vi "NI-DAQmx.vi"() -> (0 "error out":errorcluster)   [LabVIEW 2017]
uses:
  <vilib>/DAQmx/read.llb/DAQmx Read (Analog 2D DBL NChan NSamp).vi
  Globals/Meas_global.vi
  PWA/PWAtasksGLOBAL.vi
  <vilib>/DAQmx/miscellaneous.llb/DAQmx Fill In Error Info.vi
  <vilib>/DAQmx/configure/timing.llb/DAQmx Timing (Sample Clock).vi
  <vilib>/DAQmx/create/channels.llb/DAQmx Create Channel (AI-Voltage-Basic).vi
  <vilib>/Analysis/baseanly.llb/Mean (DBL).vi
  <resource>/objmgr/daqmx.rc
  <vilib>/Analysis/NI_AALBase.lvlib
panel:
  out "AuditTrail":string[](array[string])
  out "input terminal configuration":i32(ring)=10106 items=["default"=-1, "RSE"=10083, "NRSE"=10078, "Differential"=10106, "Pseudodifferential"=12529]
  out "AI.Voltage.Rngs":dbl[](array[numeric])=[-10.0, 10.0]
  out "TotalSampPerChanAcquired":dbl=1024.0
  out "AvailSampPerChan":u32
  out "CurrReadPos":dbl=1024.0
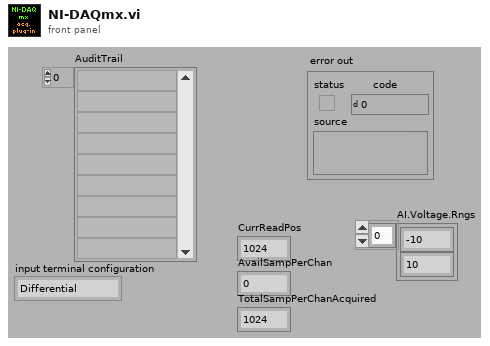
[diagram p1: front panel]
types:
  T1 = typedef "Analysis_info_cluster.ctl" = cluster{"Colour":u32, "Inst type":T2, "Inst name":string, "Symbol":string, "Code name":string, "Extra Info":string, "Inst Array":T3, "Extra Titles":string[], "Extra Values":string[], "U":dbl, "u^2":dbl, "u^3":dbl, "u^4":dbl, "Skew_u":dbl, "Kurt_u":dbl, "Sd Error in Mean":dbl, "% u'/U":dbl, "X":dbl, "Y":dbl, "Z":dbl, "Timescale integral Estimate":dbl, "Sd Error in Variance":dbl, "Calib File":path, "Calib Constants":dbl[], "Output Position":bool, "Full Stats":bool, "Av Sampling Rate":dbl, "Av No of Samples":dbl, "Total Meas Time (s)":dbl, "ADAM Ch Name":string, "Max value":dbl, "Min value":dbl, "Req Sample Rate Hz":dbl, "Sync Delay Time (s)":dbl, "Ch No":i16, "Device ID":string, "Use Latest Calib":bool}
  T2 = typedef "Inst_type.ctl" = enum16{"Propeller anemometer", "Raw voltage", "Pressure Transducer", "Pitot-static tube", "Preston tube", "Hot wire", "Cross wire 1", "Cross wire 2", "Generic Linear", "Generic Polynomial", "Generic BackPoly", "Fast FID", "Thermocouple", "Cold wire", "Pulsed Wire", "LDA Vel", "LDA Tran time", "LDA Arr time", "Microphone"}
  T3 = typedef "Instrument_Array.ctl" = enum16{"PWA", "LDA", "Analogue"}
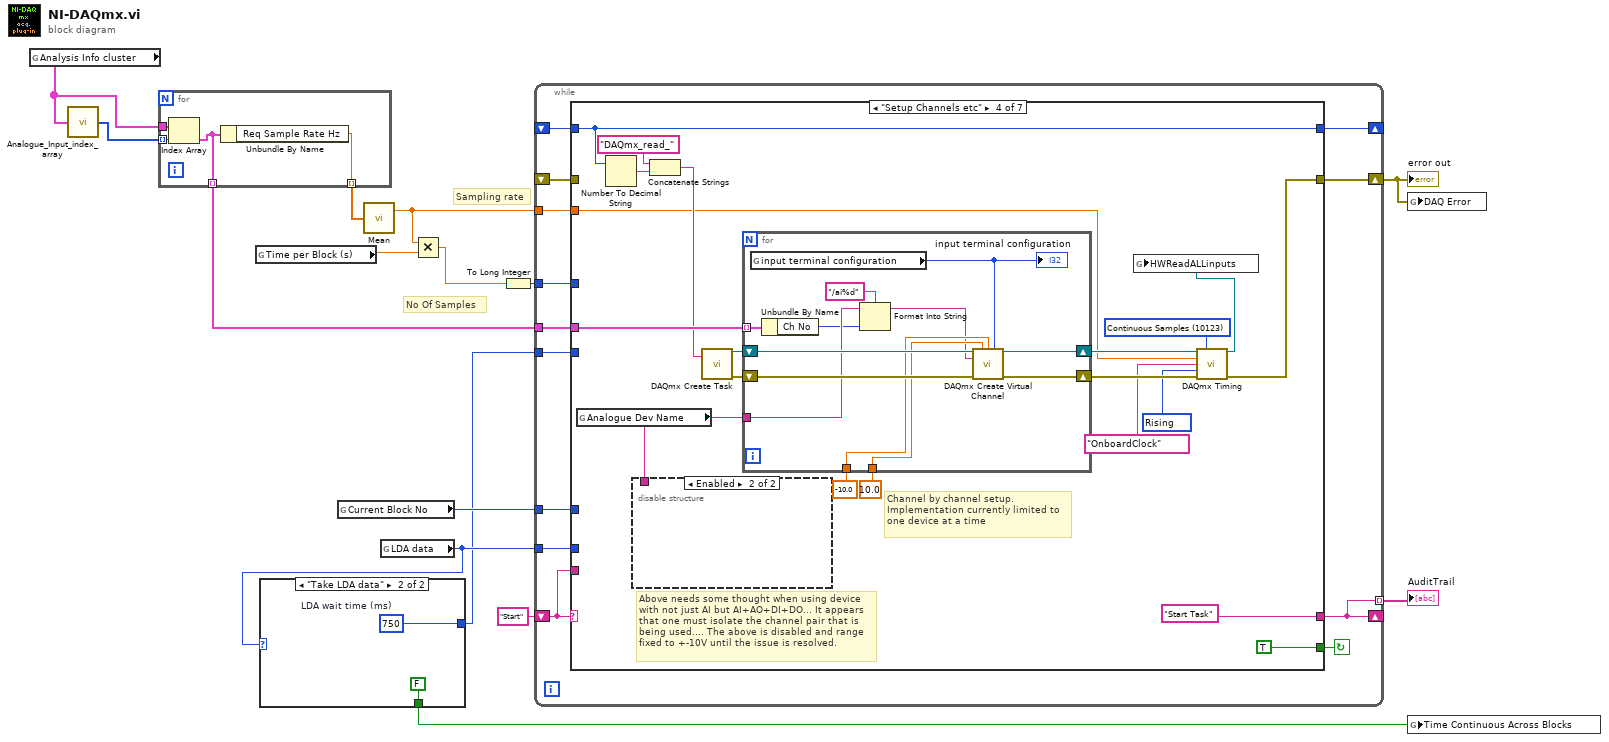
[diagram p0: block diagram]
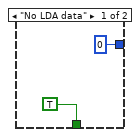
[diagram p2: hidden frame]
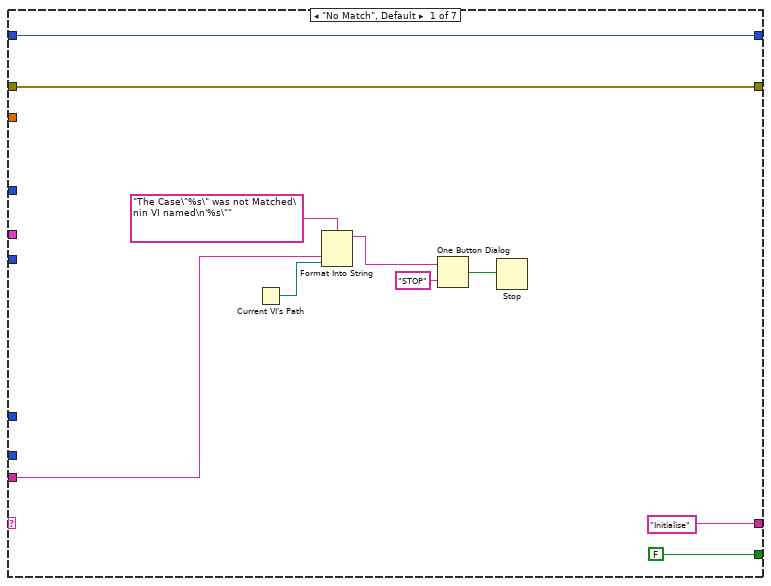
[diagram p3: hidden frame]
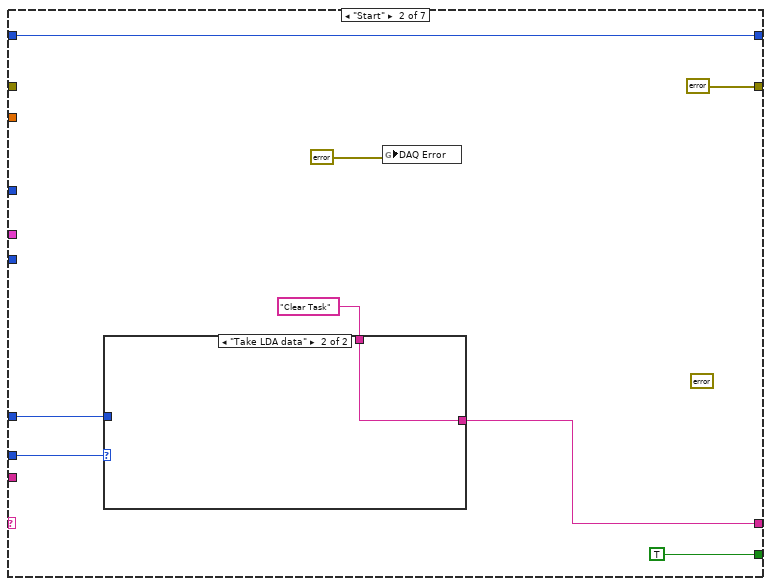
[diagram p4: hidden frame]
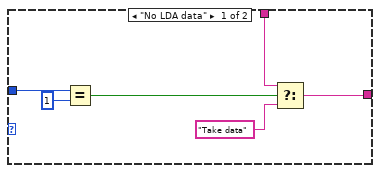
[diagram p5: hidden frame]
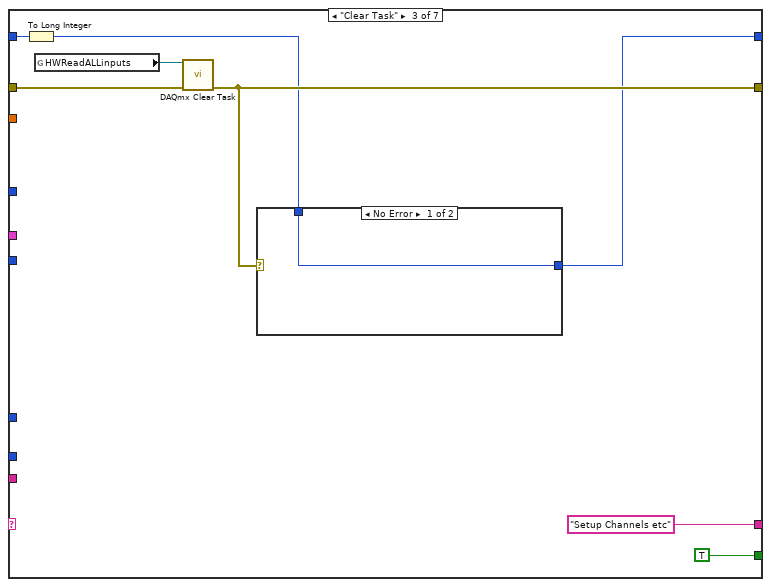
[diagram p6: hidden frame]
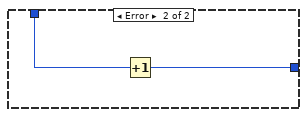
[diagram p7: hidden frame]
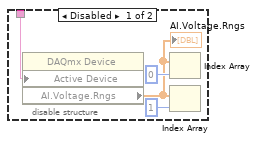
[diagram p8: hidden frame]
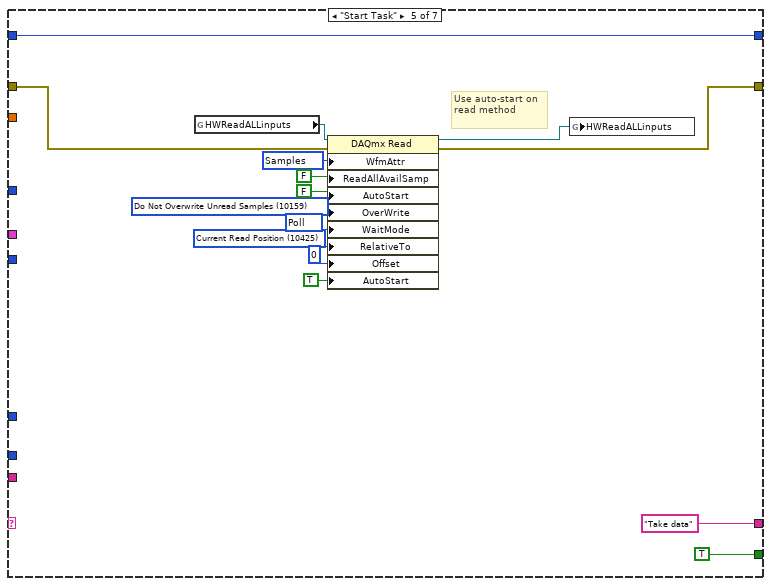
[diagram p9: hidden frame]
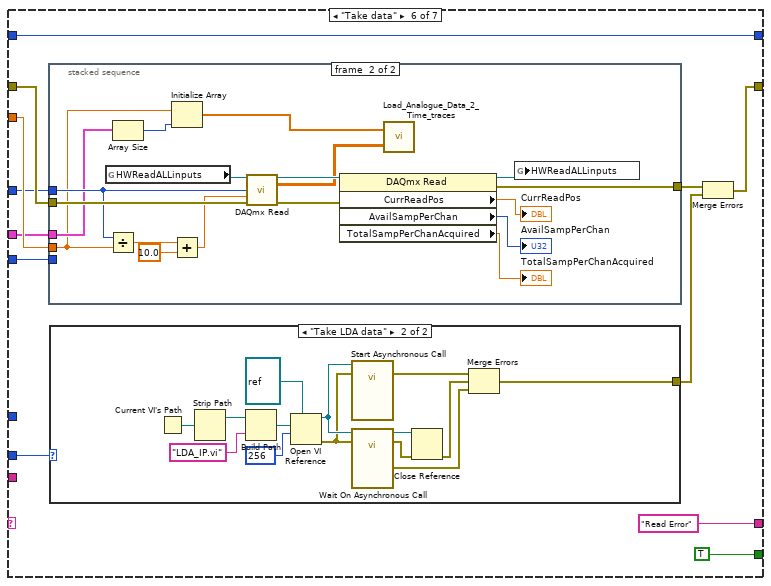
[diagram p10: hidden frame]
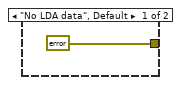
[diagram p11: hidden frame]
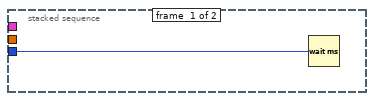
[diagram p12: hidden frame]
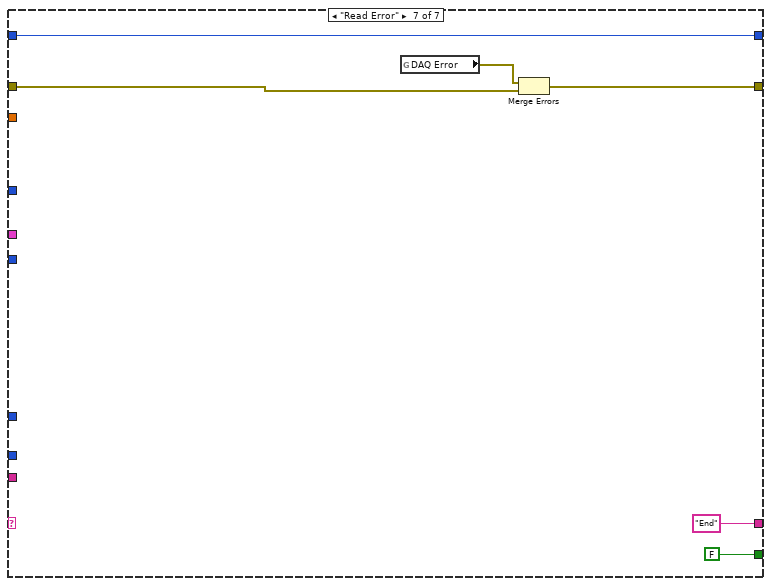
[diagram p13: hidden frame]
diagram:
  # "Sampling rate"
  # "No Of Samples"
  n1 = global read "Meas_global.vi" "Analysis Info cluster"() -> (w7:T1[])
  n2 = call "Analogue_Input_index_array.vi"("Analysis Info cluster"=w7) -> ("Array"=w2:i32[])
  n3 = for {
    tunnel: w7 -> [w19]
    tunnel: w2 -> [w18] mode=indexing
    tunnel: [w17] -> w6 mode=indexing
    tunnel: [w16] -> w1 mode=indexing
    n4 = Index Array(array=w19, index=w18) -> (element=w16:T1)
    n5 = Unbundle By Name(w16) -> ("Req Sample Rate Hz"=w17:dbl)
  }
  n6 = global read "Meas_global.vi" "Time per Block (s)"() -> (w5:dbl)
  n7 = global read "Meas_global.vi" "Current Block No"() -> (w14:i32)
  n8 = call-poly <vilib>:"Mean.vi"("X"=w6) -> ("mean"=w4:dbl)  [unwired: 1 out]
  n9 = global read "Meas_global.vi" "LDA data"() -> (w13:enum16{"No LDA data", "Take LDA data"})
  n10 = case shown="\"Take LDA data\"" w13 {
    tunnel: [TRUE ("Time Continuous across Blocks") FALSE ("Time Continuous across Blocks")] -> w10
    tunnel: [u32 0 ("LDA wait time (ms)") w22] -> w9
    frame "No LDA data" {
    }
    frame "Take LDA data" {
      w22 = u32 750  # LDA wait time (ms)
    }
  }
  n11 = Multiply(x=w4, y=w5) -> (x*y=w3:dbl)
  n12 = To Long Integer(number=w3) -> (32bit integer=w12:i32)
  n13 = while {
    shift-left: "Start" -> [w35]
    shift-right: [w25] -> _
    shift-right: [w29] -> w8
    shift-left: _ -> [w34]
    tunnel: w4 -> [w33]
    tunnel: w12 -> [w32]
    tunnel: w14 -> [w31]
    tunnel: w1 -> [w30]
    shift-right: [w28] -> _
    shift-left: _ -> [w27]
    tunnel: w13 -> [w26]
    tunnel: [w25] -> w11 mode=indexing
    tunnel: w9 -> [w24]
    stop <- w36 continue-if-true
    n14 = case shown="\"Setup Channels etc\"" w35 {
      tunnel: [FALSE TRUE TRUE TRUE TRUE TRUE FALSE] -> w36
      tunnel: ["Initialise" w52 "Setup Channels etc" "Start Task" "Take data" "Read Error" "End" ("f")] -> w25
      tunnel: w35 -> [w41 _ _ _ _ _ _]
      tunnel: [w38 errorcluster {"status"=FALSE, "code"=0, "source"=""} ("error out") w65 w86 w110 w125 w173] -> w29
      tunnel: w34 -> [w38 _ w66 _ w122 w135 w174]
      tunnel: w33 -> [_ _ _ w75 _ w131 _]
      tunnel: w32 -> [_ _ _ _ _ w130 _]
      tunnel: w31 -> [_ w49 _ _ _ _ _]
      tunnel: w30 -> [_ _ _ w85 _ w124 _]
      tunnel: [w37 w51 w64 w74 w120 w132 w172] -> w28
      tunnel: w27 -> [w37 w51 w63 w74 w120 w132 w172]
      tunnel: w26 -> [_ w48 _ _ _ w128 _]
      tunnel: w24 -> [_ _ _ _ _ w129 _]
      frame "No Match", Default {
        n15 = Current VI's Path() -> (path=w40:path)
        n16 = Format Into String(format string="The Case\"%s\" was not Matched\nin VI named\n'%s\"" ("Format String"), w41, w40) -> (resulting string=w44:string)  [unwired: 2 in, 1 out]
        n17 = One Button Dialog(message=w44, button name ("OK")="STOP") -> (true=w42:bool)
        n18 = Stop(stop? (T)=w42) -> ()
      }
      frame "Start" {
        (unwired) errorcluster {"status"=FALSE, "code"=0, "source"=""} ("error out")
        n19 = case shown="\"Take LDA data\"" w48 {
          tunnel: "Clear Task" -> [w60 w61]
          tunnel: [w58 w61] -> w52
          tunnel: w49 -> [w57 _]
          frame "No LDA data" {
            n20 = Equal?(x=w57, y=1) -> (x = y?=w55:bool)
            n21 = Select(t=w60, s=w55, f="Take data") -> (s? t:f=w58:string)
          }
          frame "Take LDA data" {
          }
        }
        n22 = global write "Meas_global.vi" "DAQ Error"(errorcluster {"status"=FALSE, "code"=0, "source"=""} ("DAQ Error")) -> ()
      }
      frame "Clear Task" {
        n23 = To Long Integer(number=w63) -> (32bit integer=w62:i32)
        n24 = global read "PWAtasksGLOBAL.vi" "HWReadALLinputs"() -> (w67:refnum<k21>)
        n25 = call <vilib>:"DAQmx Clear Task.vi"("task in"=w67, "error in"=w66) -> ("error out"=w65:errorcluster)  [unwired: 13 out]
        n26 = case shown="No Error" w65 {
          tunnel: [w70 w71] -> w64
          tunnel: w62 -> [w70 w72]
          frame No Error {
          }
          frame Error {
            n27 = Increment(x=w72) -> (x+1=w71:i32)
          }
        }
      }
      frame "Setup Channels etc" {
        w83 = 10280 items=["Rising"=10280, "Falling"=10171] ("active edge")
        w89 = 10123 items=["Finite Samples"=10178, "Continuous Samples"=10123, "Hardware Timed Single Point"=12522] ("sample mode")
        # "Above needs some thought when using device with not just AI but AI+AO+DI+DO... It appears that one must isolate the channel pair that is being used.... The above is disabled and range fixed to +-10V until the issue is resolved."
        # "Channel by channel setup. Implementation currently limited to one device at a time"
        n28 = global read "PWAtasksGLOBAL.vi" "Analogue Dev Name"() -> (w78:string)
        n29 = Number To Decimal String(number=w74) -> (decimal integer string=w73:string)  [unwired: 1 in]
        n30 = disable-structure shown="Enabled" {
          disable-tunnel: w78 -> [w93 _]
          frame Disabled {
            n31 = property class="DAQmx Device"("Active Device"=w93) -> ("AI.Voltage.Rngs"=w94:dbl[])  [unwired: 2 in, 2 out]
            "AI.Voltage.Rngs" <- w94
            n32 = Index Array(array=w94, index=0) -> ()  [unwired: 1 out]
            n33 = Index Array(array=w94, index=1) -> ()  [unwired: 1 out]
          }
          frame Enabled {
          }
        }
        n34 = Concatenate Strings("DAQmx_read_" ("new task name"), w73) -> (w76:string)
        n35 = call <vilib>:"DAQmx Create Task.vi"("new task name"=w76) -> ("task out"=w87:refnum<k21>, "error out"=w90:errorcluster)  [unwired: 4 in, 9 out]
        n36 = for {
          tunnel: w85 -> [w108] mode=indexing
          shift-right: [w106] -> w88
          shift-left: w87 -> [w107]
          shift-right: [w104] -> w91
          shift-left: w90 -> [w105]
          tunnel: w78 -> [w101]
          tunnel: -10.0 -> [w103]
          tunnel: 10.0 -> [w102]
          n37 = global read "Meas_global.vi" "input terminal configuration"() -> (w97:i32)
          "input terminal configuration" <- w97
          n38 = Unbundle By Name(w108) -> ("Ch No"=w100:i16)
          n39 = Format Into String(format string="/ai%d", initial string=w101, w100) -> (resulting string=w98:string)  [unwired: 1 in, 1 out]
          n40 = call-poly <vilib>:"DAQmx Create Virtual Channel.vi"("task in"=w107, "maximum value"=w102, "minimum value"=w103, "input terminal configuration"=w97, "physical channels"=w98, "error in"=w105) -> ("task out"=w106:refnum<k21>, "error out"=w104:errorcluster)  [unwired: 3 in, 5 out]
        }
        n41 = call-poly <vilib>:"DAQmx Timing.vi"("task/channels in"=w88, "sample mode"=w89, "rate"=w75, "source"=tag "OnboardClock", "active edge"=w83, "error in"=w91) -> ("task out"=w84:refnum<k21>, "error out"=w86:errorcluster)  [unwired: 1 in, 7 out]
        n42 = global write "PWAtasksGLOBAL.vi" "HWReadALLinputs"(w84) -> ()
      }
      frame "Start Task" {
        w114 = 10425 items=["First Sample"=10424, "Current Read Position"=10425, "Reference Trigger"=10426, "First Pretrigger Sample"=10427, "Most Recent Sample"=10428] ("RelativeTo")
        w115 = 12524 items=["Wait For Interrupt"=12523, "Poll"=12524, "Yield"=12525, "Sleep"=12547] ("WaitMode")
        w116 = 10159 items=["Overwrite Unread Samples"=10252, "Do Not Overwrite Unread Samples"=10159] ("OverWrite")
        w118 = 10287 items=["Samples"=10287, "Samples and Timing"=10140, "Samples, Timing, and Attributes"=10141] ("WfmAttr")
        # "Use auto-start on read method"
        n43 = global read "PWAtasksGLOBAL.vi" "HWReadALLinputs"() -> (w112:refnum<k21>)
        n44 = property class="DAQmx Read"(reference=w112, error in=w122, "WfmAttr"=w118, "ReadAllAvailSamp"=FALSE, "AutoStart"=FALSE, "OverWrite"=w116, "WaitMode"=w115, "RelativeTo"=w114, "Offset"=0, "AutoStart"=TRUE) -> (reference out=w111:refnum<k21>, error out=w110:errorcluster)
        n45 = global write "PWAtasksGLOBAL.vi" "HWReadALLinputs"(w111) -> ()
      }
      frame "Take data" {
        n46 = stacked-sequence {
          tunnel: w135 -> [_ w169]
          tunnel: w131 -> [_ w153]
          tunnel: w130 -> [_ w158]
          tunnel: [_ w157] -> w126
          tunnel: w129 -> [w151 _]
          tunnel: w124 -> [_ w155]
          frame #0 {
            n47 = Wait (ms)(milliseconds to wait=w151) -> ()  [unwired: 1 out]
          }
          frame #1 {
            n48 = global read "PWAtasksGLOBAL.vi" "HWReadALLinputs"() -> (w163:refnum<k21>)
            n49 = Divide(x=w158, y=w153) -> (x/y=w161:dbl)
            n50 = Array Size(array=w155) -> (size(s)=w154:i32)
            n51 = Initialize Array(w153, w154) -> (w152:dbl[])
            n52 = Add(x=w161, y=10.0) -> (x+y=w159:dbl)
            n53 = call-poly <vilib>:"DAQmx Read.vi"("task/channels in"=w163, "number of samples per channel"=w158, "timeout"=w159, "error in"=w169) -> ("task out"=w166:refnum<k21>, "data"=w156:dbl[][], "error out"=w162:errorcluster)  [unwired: 9 out]
            n54 = property class="DAQmx Read"(reference=w166, error in=w162) -> (reference out=w165:refnum<k21>, error out=w157:errorcluster, "CurrReadPos"=→"CurrReadPos":dbl, "AvailSampPerChan"=→"AvailSampPerChan":u32, "TotalSampPerChanAcquired"=→"TotalSampPerChanAcquired":dbl)
            n55 = call "Load_Analogue_Data_2_Time_traces.vi"("Voltage Array"=w156, "Sampling Rate (Hz)"=w152) -> ()  [unwired: 1 in]
            n56 = global write "PWAtasksGLOBAL.vi" "HWReadALLinputs"(w165) -> ()
          }
        }
        n57 = case shown="\"Take LDA data\"" w128 {
          tunnel: [errorcluster {"status"=FALSE, "code"=0, "source"=""} ("error out") w137] -> w127
          frame "No LDA data", Default {
          }
          frame "Take LDA data" {
            n58 = Current VI's Path() -> (path=w148:path)
            n59 = Strip Path(path=w148) -> (stripped path=w147:path)  [unwired: 1 out]
            n60 = Build Path(base path=w147, name or relative path="LDA_IP.vi") -> (appended path=w149:path)
            n61 = Open VI Reference(type specifier VI Refnum (for type only)=refnum<vi> refnum, vi path=w149, options=256) -> (vi reference=w144:refnum<vi>, error out=w143:errorcluster)  [unwired: 3 in]
            n62 = call-by-ref "Start Asynchronous Call"(reference=w144, error in=w143) -> (error out=w140:errorcluster)  [unwired: 1 in, 2 out]
            n63 = call-by-ref "Wait On Asynchronous Call"(reference=w144, error in=w143) -> (reference out=w142:refnum<vi>, error out=w141:errorcluster, 0:"error out"=w138:errorcluster)  [unwired: 1 in]
            n64 = Close Reference(reference=w142, error in (no error)=w141) -> (error out=w139:errorcluster)
            n65 = Merge Errors(w140, w139, w138) -> (w137:errorcluster)
          }
        }
        n66 = Merge Errors(w126, w127) -> (w125:errorcluster)
      }
      frame "Read Error" {
        n67 = global read "Meas_global.vi" "DAQ Error"() -> (w175:errorcluster)
        n68 = Merge Errors(w175, w174) -> (w173:errorcluster)
      }
    }
  }
  "error out" <- w8
  "AuditTrail" <- w11
  n69 = global write "Meas_global.vi" "DAQ Error"(w8) -> ()
  n70 = global write "Meas_global.vi" "Time Continuous Across Blocks"(w10) -> ()
